vi "GetAll.vi"() -> (2 "DebugHandles":refnum<class "DebugTraceHandle.lvclass">[](array[class]))   [LabVIEW 2024, in "DebugTraceSingleton.lvlib"]
uses:
  DebugTraceSingleton.lvlib
  DebugTraceHandle/DebugTraceHandle.lvclass
  Command.ctl
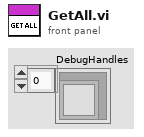
[diagram p1: front panel]
types:
  T1 = typedef "DebugTraceSingleton.lvlib/Command.ctl" = enum16{"Add", "Remove", "Get", "GetAll"}
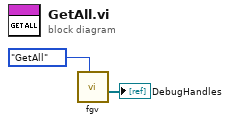
[diagram p0: block diagram]
diagram:
  n1 = call "fgv.vi"("Command"=Command."GetAll") -> ("Array"=→"DebugHandles":refnum<class "DebugTraceHandle.lvclass">[])  [unwired: 8 in, 2 out]
